vi "Puff_release2_chs.vi"() -> (5 "Plug in titles":string[](array[string]), 7 "Plug in values":string[](array[string]))   [LabVIEW 2010]
uses:
  Controls/Post_Process.ctl
  Globals/Plug_in_data_global.vi
  Globals/Meas_global.vi
  Globals/Constants_global.vi
  Globals/Dynamic_call_global.ph.vi
  <vilib>/Analysis/NI_AALPro.lvlib
panel:
  in  "PDF samples per block\n(after downsampling)":i32
  in  "Output Directory":path
  in  "Per Block Mode":T1(ring)
  in  "Averaging Samples":i32=1 min=1
  out "Valve trigger Index":dbl format="%.2f"
  out "delay":dbl format="%.2f"
  out "Pulse Width":dbl format="%.2f"
  out "falltime":dbl format="%.2f"
  out "top":dbl format="%.2f"
  out "risetime":dbl format="%.2f"
  in  "Save Time pdf?":bool
  out "Pdf":cluster{"Axis":dbl[], dbl[]}(graph)
  in  "PDF start time (s)":dbl format="%.2f"
  out "Current Block No":i32
  in  "Save averaged traces?":bool
  in  "Pause Mode":T2(ring)
  in  "OK":bool
  out "No of Valid Blocks":dbl
  out "Valve Trace":dbl[](graph)
  out "FFID Trace":cluster{dbl, dbl, dbl[]}(graph)
  out "Valve On":i32
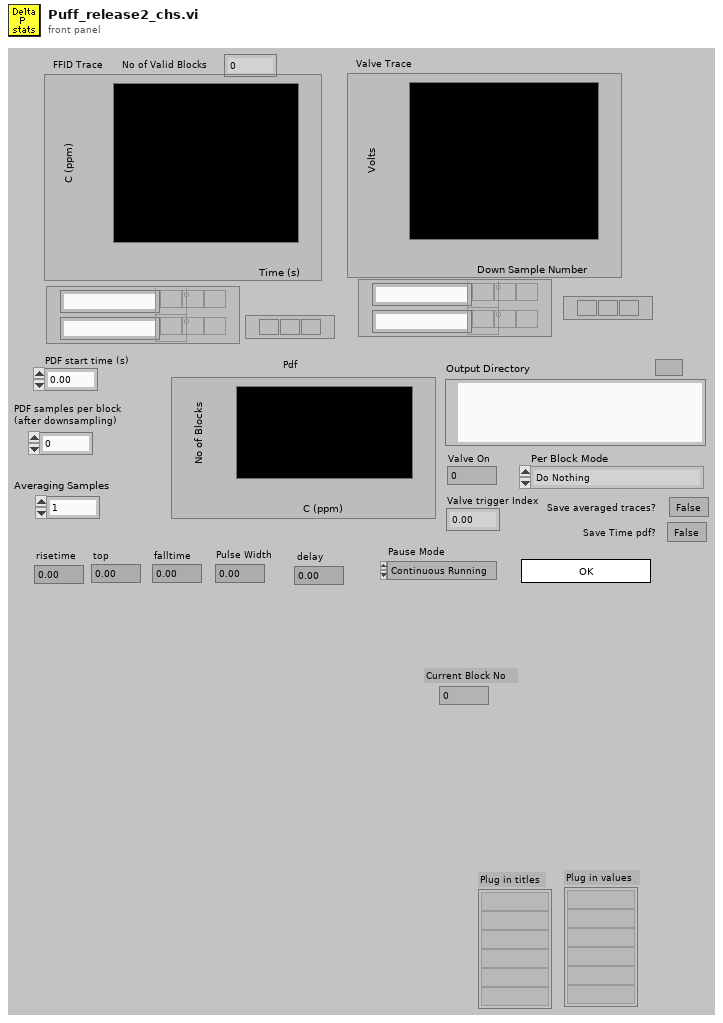
[diagram p1: front panel]
types:
  T1 = enum16{"Do Nothing", "Save Block Time Traces", "Save Jpeg plots"}
  T2 = enum16{"Continuous Running", "After Each  Block"}
  T3 = typedef "Post_Process.ctl" = enum16{"Take New Data", "Post Process Raw Data File"}
  T4 = enum32{"existing file", "new file", "new or existing file", "existing dir", "new dir", "new or existing dir", "existing file (use LLBs)", "new file (use LLBs)", "new or existing file (use LLBs)", "new or existing file or directory (use LLBs)"}
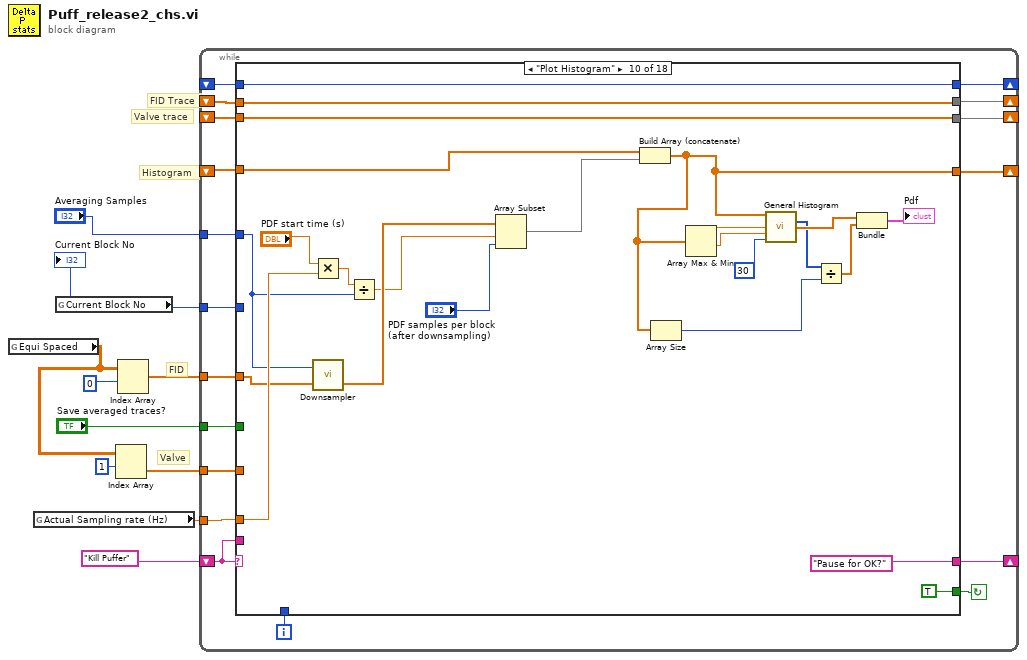
[diagram p0: block diagram]
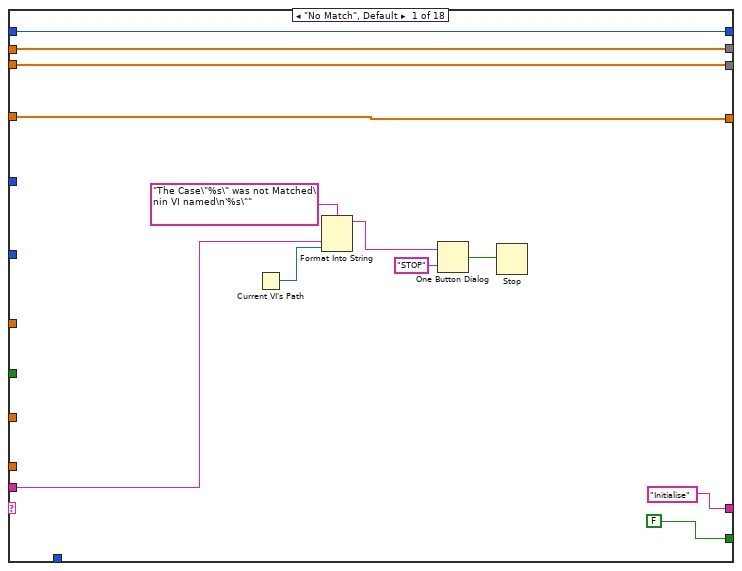
[diagram p2: hidden frame]
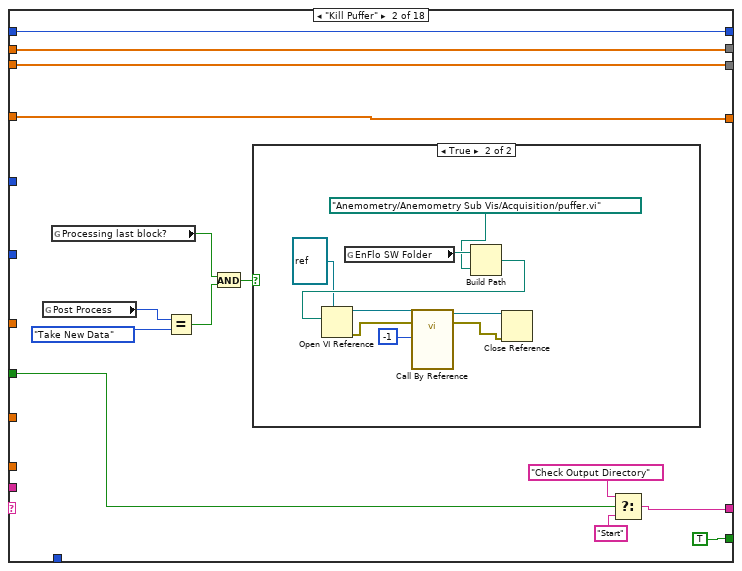
[diagram p3: hidden frame]
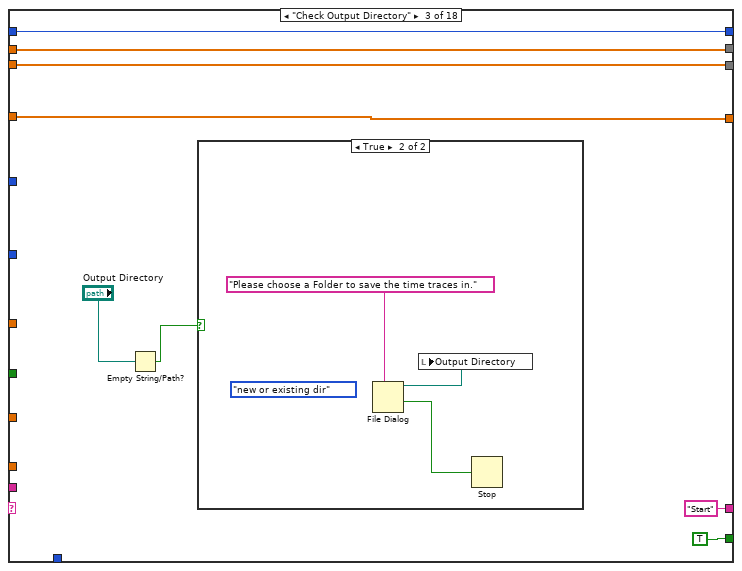
[diagram p5: hidden frame]
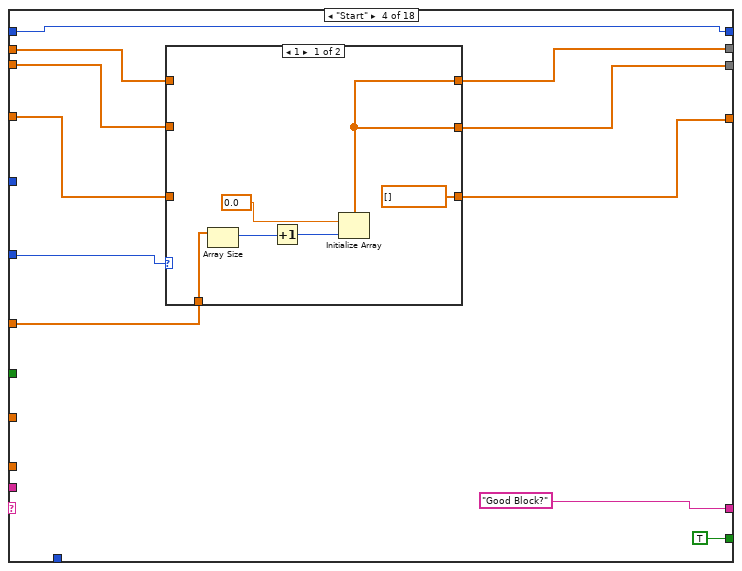
[diagram p7: hidden frame]
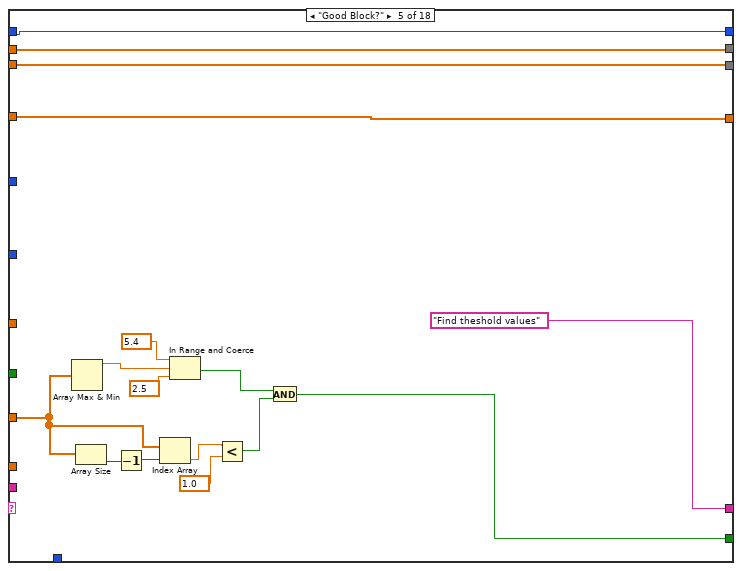
[diagram p9: hidden frame]
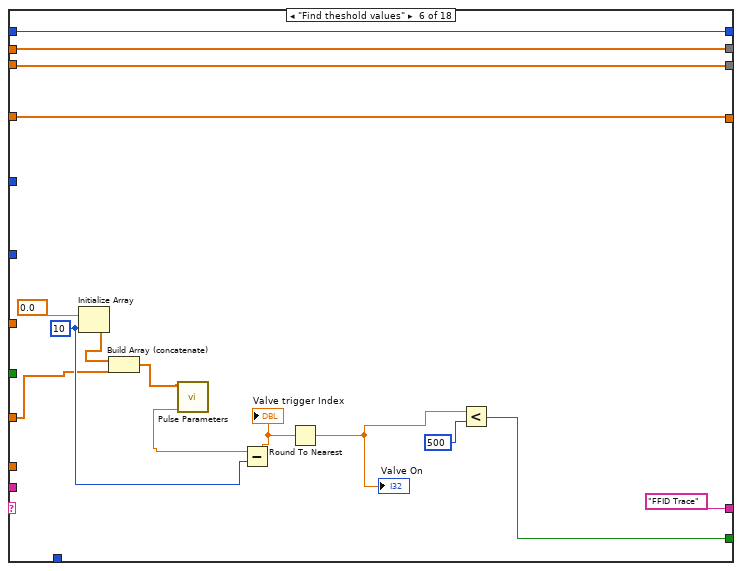
[diagram p10: hidden frame]
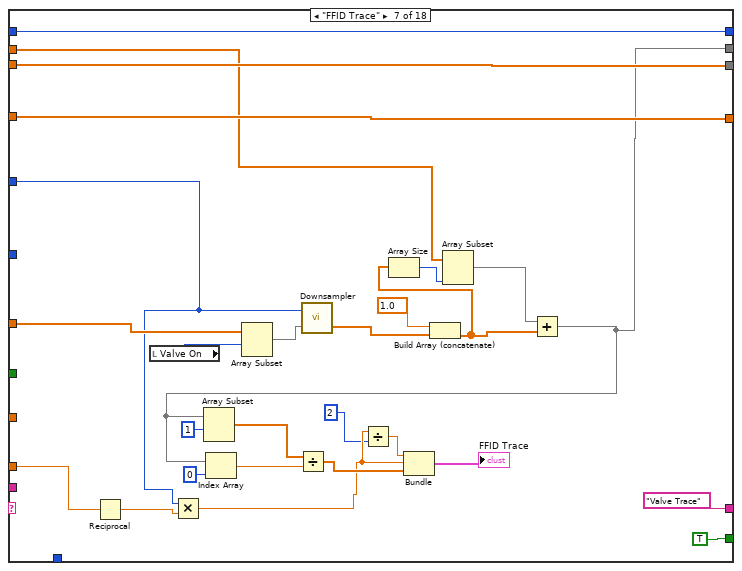
[diagram p11: hidden frame]
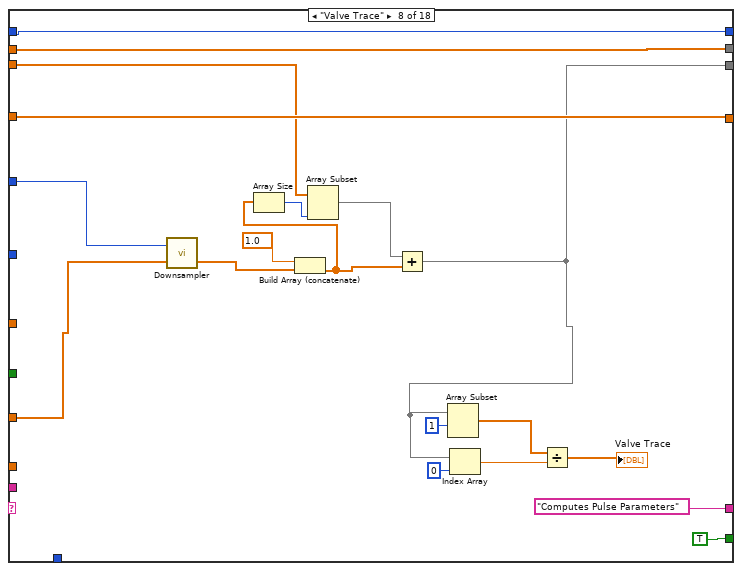
[diagram p12: hidden frame]
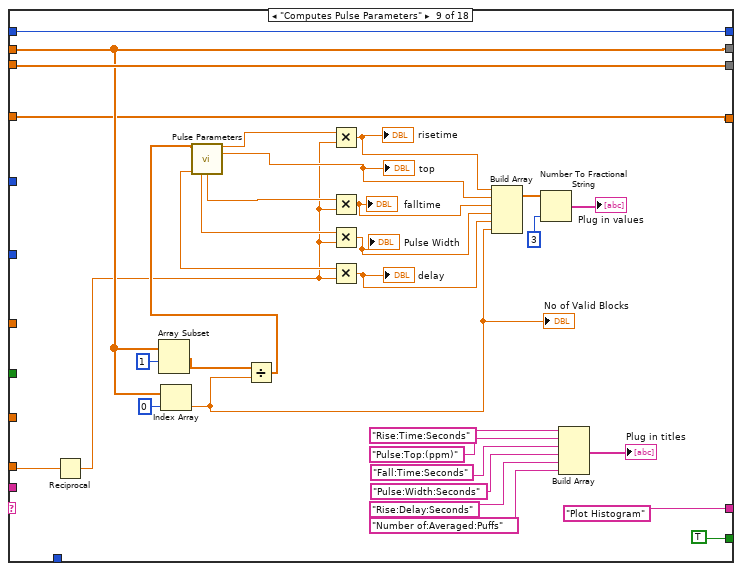
[diagram p13: hidden frame]
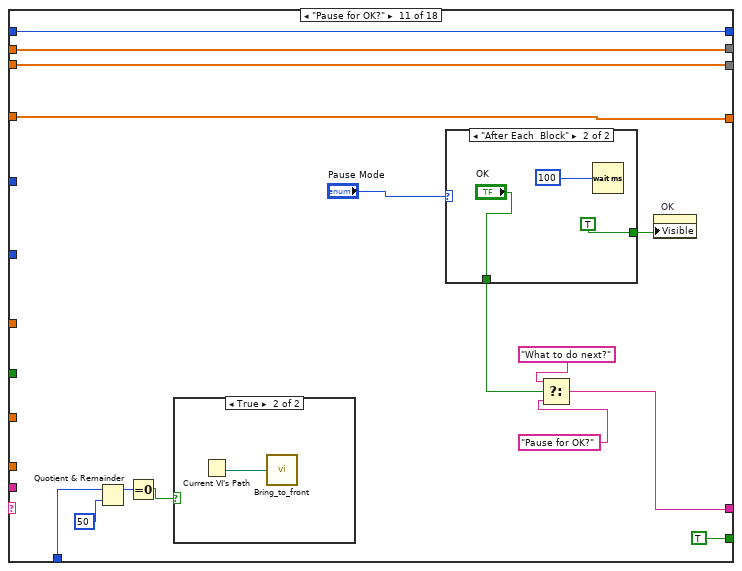
[diagram p14: hidden frame]
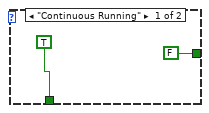
[diagram p16: hidden frame]
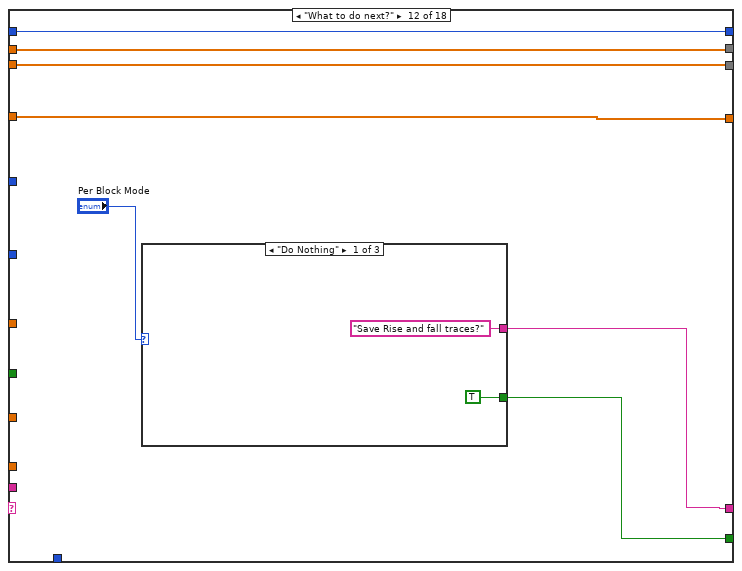
[diagram p17: hidden frame]
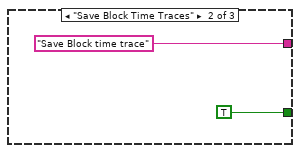
[diagram p18: hidden frame]
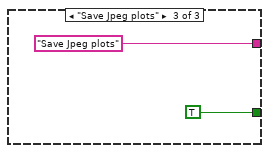
[diagram p19: hidden frame]
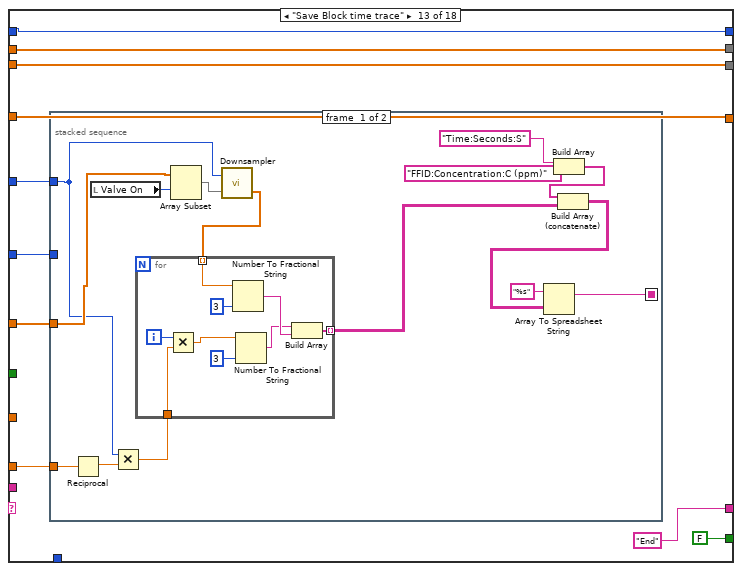
[diagram p20: hidden frame]
diagram:
  # "Valve"
  # "FID"
  # "Histogram"
  # "Valve trace"
  # "FID Trace"
  n1 = global read "Plug_in_data_global.vi" "Equi Spaced"() -> (w5:dbl[][])
  n2 = global read "Meas_global.vi" "Actual Sampling rate (Hz)"() -> (w8:dbl)
  n3 = global read "Meas_global.vi" "Current Block No"() -> (w7:i32)
  "Current Block No" <- w7
  n4 = Index Array(array=w5, index (row)=1) -> (element=w4:dbl[])  [unwired: 1 in]
  n5 = Index Array(array=w5, index (row)=0) -> (element=w9:dbl[])  [unwired: 1 in]
  n6 = while {
    shift-left: "Kill Puffer" -> [w26]
    shift-right: [w27] -> _
    shift-right: [w25] -> _
    shift-left: _ -> [w22]
    shift-right: [w24] -> _
    shift-left: _ -> [w23]
    tunnel: w9 -> [w21]
    tunnel: w8 -> [w20]
    tunnel: w7 -> [w19]
    shift-right: [w16] -> _
    shift-left: _ -> [w17]
    shift-right: [w14] -> _
    shift-left: _ -> [w15]
    tunnel: w4 -> [w13]
    tunnel: "Averaging Samples" -> [w12]
    tunnel: "Save averaged traces?" -> [w11]
    i -> [w18]
    stop <- w28 continue-if-true
    n7 = case shown="\"Plot Histogram\"" w26 {
      tunnel: [FALSE TRUE ("Processing last block?") TRUE ("Processing last block?") TRUE ("Processing last block?") w99 w121 TRUE ("Processing last block?") TRUE ("Processing last block?") TRUE ("Processing last block?") TRUE ("Processing last block?") TRUE ("Processing last block?") w249 FALSE ("Processing last block?") FALSE ("Processing last block?") w318 TRUE ("Processing last block?") "Save Time pdf?" FALSE ("Processing last block?")] -> w28
      tunnel: ["Initialise" w41 "Start" "Good Block?" "Find theshold values" "FFID Trace" "Valve Trace" "Computes Pulse Parameters" "Plot Histogram" ("f") "Pause for OK?" ("f") w230 w250 "End" "End" w320 "Save Time pdf?" "Save Time pdf" "End"] -> w27
      tunnel: w26 -> [w35 _ _ _ _ _ _ _ _ _ _ _ _ _ _ _ _ _]
      tunnel: [w32 w54 w71 w84 w110 w124 w141 w169 w174 w227 w242 w255 w271 w316 w325 w332 w407 w415] -> w25
      tunnel: [w31 w53 w70 w82 w109 w123 w150 w153 w201 w226 w241 w254 w270 w315 w324 w331 w406 w414] -> w24
      tunnel: w23 -> [w31 w53 w70 w81 w109 w123 w150 w154 w201 w226 w241 w254 w270 w315 w324 w331 w406 w414]
      tunnel: w22 -> [w32 w54 w71 w83 w110 w124 w130 w169 w174 w227 w242 w255 w271 w316 w325 w332 w407 w415]
      tunnel: w21 -> [_ _ _ w80 _ _ w149 _ _ w208 _ _ w267 w310 _ _ _ w411]
      tunnel: w20 -> [_ _ _ _ _ _ w138 _ w199 w223 _ _ w262 w307 _ _ _ _]
      tunnel: w19 -> [_ _ _ w79 _ _ _ _ _ _ _ _ w266 _ _ _ _ w410]
      tunnel: w18 -> [_ _ _ _ _ _ _ _ _ _ w239 _ _ _ _ _ _ _]
      tunnel: w17 -> [w30 w51 w67 w76 w100 w120 w146 w168 w197 w225 w235 w253 w265 w312 _ w328 _ w409]
      tunnel: [w30 w51 w67 w76 w100 w120 w146 w168 w197 w225 w235 w253 w265 w312 0 w328 0 w409] -> w16
      tunnel: w15 -> [w29 w48 w66 w77 w98 w115 w145 w163 w173 w221 w234 w252 w264 w311 w319 w327 w402 w408]
      tunnel: [w29 w48 w66 w78 w98 w115 w145 w163 w173 w213 w234 w252 w264 w311 w319 w327 w402 w408] -> w14
      tunnel: w13 -> [_ _ _ _ w95 w112 _ w156 _ _ _ _ _ _ _ _ _ _]
      tunnel: w12 -> [_ _ _ _ _ _ w135 w155 _ w205 _ _ w263 _ _ w326 _ _]
      tunnel: w11 -> [_ w44 _ _ _ _ _ _ _ _ _ _ _ _ w317 _ _ _]
      frame "No Match", Default {
        n8 = Current VI's Path() -> (path=w34:path)
        n9 = Format Into String(format string="The Case\"%s\" was not Matched\nin VI named\n'%s\"" ("Format String"), w35, w34) -> (resulting string=w38:string)  [unwired: 2 in, 1 out]
        n10 = One Button Dialog(message=w38, button name ("OK")="STOP") -> (true=w36:bool)
        n11 = Stop(stop? (T)=w36) -> ()
      }
      frame "Kill Puffer" {
        n12 = global read "Meas_global.vi" "Post Process"() -> (w50:T3)
        n13 = global read "Meas_global.vi" "Processing last block?"() -> (w46:bool)
        n14 = Equal?(x=w50, y=Post_Process."Take New Data" ("Post Process")) -> (x = y?=w47:bool)
        n15 = And(x=w46, y=w47) -> (x .and. y?=w45:bool)
        n16 = case shown="True" w45 {
          frame False {
          }
          frame True {
            n17 = global read "Constants_global.vi" "EnFlo SW Folder"() -> (w63:path)
            n18 = Build Path(base path=w63, name or relative path=path "Anemometry/Anemometry Sub Vis/Acquisition/puffer.vi") -> (appended path=w61:path)
            n19 = Open VI Reference(type specifier VI Refnum (for type only)=refnum<vi> refnum, vi path=w61) -> (vi reference=w60:refnum<vi>, error out=w56:errorcluster)  [unwired: 1 in, 3 out]
            n20 = call-by-ref "?"(reference=w60, error in=w56, "number of puffs (cont:0, stop:-1)"=-1) -> (reference out=w57:refnum<vi>, error out=w55:errorcluster)  [unwired: 2 in, 2 out]
            n21 = Close Reference(reference=w57, error in (no error)=w55) -> ()  [unwired: 1 out]
          }
        }
        n22 = Select(t="Check Output Directory", s=w44, f="Start") -> (s? t:f=w41:string)
      }
      frame "Check Output Directory" {
        n23 = Empty String/Path?(string/path="Output Directory") -> (empty?=w65:bool)
        n24 = case shown="True" w65 {
          frame False {
          }
          frame True {
            (unwired) T4."new or existing dir" ("select mode (2)")
            n25 = File Dialog(7:"Please choose a Folder to save the time traces in." ("prompt")) -> (1:w73:bool, 3:w74:path)  [unwired: 1 in, 7 out]
            n26 = local write "Output Directory"(w74) -> ()
            n27 = Stop(stop? (T)=w73) -> ()
          }
        }
      }
      frame "Start" {
        n28 = case shown="1" w79 {
          tunnel: [w87 w94] -> w84
          tunnel: w83 -> [_ w94]
          tunnel: [w87 w93] -> w82
          tunnel: w81 -> [_ w93]
          tunnel: w80 -> [w91 _]
          tunnel: [dbl[] [] w92] -> w78
          tunnel: w77 -> [_ w92]
          frame 1 {
            n29 = Array Size(array=w91) -> (size(s)=w90:i32)
            n30 = Increment(x=w90) -> (x+1=w86:i32)
            n31 = Initialize Array(0.0 ("element"), w86) -> (w87:dbl[])
          }
          frame 2, Default {
          }
        }
      }
      frame "Good Block?" {
        n32 = Array Max & Min(array=w95) -> (max value=w97:dbl)  [unwired: 3 out]
        n33 = Array Size(array=w95) -> (size(s)=w106:i32)
        n34 = Decrement(x=w106) -> (x-1=w105:i32)
        n35 = Index Array(array=w95, index=w105) -> (element=w104:dbl)
        n36 = In Range and Coerce(upper limit=5.4, x=w97, lower limit=2.5 ("y")) -> (In Range?=w101:bool)  [unwired: 1 out]
        n37 = Less?(x=w104, y=1.0) -> (x < y?=w102:bool)
        n38 = And(x=w101, y=w102) -> (x .and. y?=w99:bool)
      }
      frame "Find theshold values" {
        w116 = 10 ("dimension size")
        n39 = Initialize Array(0.0, w116) -> (w117:dbl[])
        n40 = Build Array (concatenate)(w117, w112) -> (w118:dbl[])
        n41 = call <vilib>:"Pulse Parameters.vi"("X"=w118) -> ("delay"=w114:dbl)  [unwired: 14 out]
        n42 = Subtract(x=w114, y=w116) -> (x-y=w113:dbl)
        "Valve trigger Index" <- w113
        n43 = Round To Nearest(number=w113) -> (nearest integer value=w111:dbl)
        "Valve On" <- w111
        n44 = Less?(x=w111, y=500) -> (x < y?=w121:bool)
      }
      frame "FFID Trace" {
        n45 = Reciprocal(x=w138) -> (1/x=w134:dbl)
        n46 = local read "Valve On"() -> (w147:i32)
        n47 = Multiply(x=w135, y=w134) -> (x*y=w128:dbl)
        n48 = Array Subset(array=w149, index=w147) -> (w136:dbl[])  [unwired: 1 in]
        n49 = call "Downsampler.vi"("Input Array"=w136, "Averaging samples"=w135) -> ("Downsampled Array"=w133:dbl[])  [unwired: 1 out]
        n50 = Divide(x=w128, y=2) -> (x/y=w126:dbl)
        n51 = Build Array (concatenate)(1.0, w133) -> (w131:dbl[])
        n52 = Array Size(array=w131) -> (size(s)=w132:i32)
        n53 = Array Subset(array=w130, length=w132) -> (w129:dbl[])  [unwired: 1 in]
        n54 = Add(x=w129, y=w131) -> (x+y=w141:dbl[])
        n55 = Array Subset(array=w141, index=1) -> (w140:dbl[])  [unwired: 1 in]
        n56 = Index Array(array=w141, index=0) -> (element=w139:dbl)
        n57 = Divide(x=w140, y=w139) -> (x/y=w144:dbl[])
        n58 = Bundle(w126, w128, w144) -> (→"FFID Trace":cluster{dbl, dbl, dbl[]})  [unwired: 1 out]
      }
      frame "Valve Trace" {
        n59 = call "Downsampler.vi"("Input Array"=w156, "Averaging samples"=w155) -> ("Downsampled Array"=w160:dbl[])  [unwired: 1 out]
        n60 = Build Array (concatenate)(1.0, w160) -> (w158:dbl[])
        n61 = Array Size(array=w158) -> (size(s)=w159:i32)
        n62 = Array Subset(array=w154, length=w159) -> (w157:dbl[])  [unwired: 1 in]
        n63 = Add(x=w157, y=w158) -> (x+y=w153:dbl[])
        n64 = Array Subset(array=w153, index=1) -> (w165:dbl[])  [unwired: 1 in]
        n65 = Index Array(array=w153, index=0) -> (element=w164:dbl)
        n66 = Divide(x=w165, y=w164) -> (x/y=→"Valve Trace":dbl[])
      }
      frame "Computes Pulse Parameters" {
        n67 = Reciprocal(x=w199) -> (1/x=w172:dbl)
        n68 = Array Subset(array=w174, index=1) -> (w177:dbl[])  [unwired: 1 in]
        n69 = Index Array(array=w174, index=0) -> (element=w176:dbl)
        "No of Valid Blocks" <- w176
        n70 = Divide(x=w177, y=w176) -> (x/y=w175:dbl[])
        n71 = call <vilib>:"Pulse Parameters.vi"("X"=w175) -> ("risetime"=w196:dbl, "top"=w182:dbl, "delay"=w193:dbl, "duration"=w194:dbl, "falltime"=w195:dbl)  [unwired: 10 out]
        "top" <- w182
        n72 = Multiply(x=w196, y=w172) -> (x*y=w181:dbl)
        "risetime" <- w181
        n73 = Multiply(x=w195, y=w172) -> (x*y=w180:dbl)
        "falltime" <- w180
        n74 = Multiply(x=w194, y=w172) -> (x*y=w179:dbl)
        "Pulse Width" <- w179
        n75 = Multiply(x=w193, y=w172) -> (x*y=w178:dbl)
        "delay" <- w178
        n76 = Build Array(w181, w182, w180, w179, w178, w176) -> (w192:dbl[])
        n77 = Number To Fractional String(number=w192, precision (6)=i16 3) -> (F-format string=→"Plug in values":string[])  [unwired: 2 out]
        n78 = Build Array("Rise:Time:Seconds", "Pulse:Top:(ppm)", "Fall:Time:Seconds", "Pulse:Width:Seconds", "Rise:Delay:Seconds", "Number of:Averaged:Puffs") -> (→"Plug in titles":string[])
      }
      frame "Plot Histogram" {
        n79 = Multiply(x="PDF start time (s)", y=w223) -> (x*y=w206:dbl)
        n80 = call "Downsampler.vi"("Input Array"=w208, "Averaging samples"=w205) -> ("Downsampled Array"=w207:dbl[])  [unwired: 1 out]
        n81 = Divide(x=w206, y=w205) -> (x/y=w204:dbl)
        n82 = Array Subset(array=w207, index=w204, length="PDF samples per block\n(after downsampling)") -> (w222:dbl[])
        n83 = Build Array (concatenate)(w221, w222) -> (w213:dbl[])
        n84 = Array Size(array=w213) -> (size(s)=w211:i32)
        n85 = Array Max & Min(array=w213) -> (max value=w220:dbl, min value=w219:dbl)  [unwired: 2 out]
        n86 = call <vilib>:"General Histogram.vi"("X"=w213, "max"=w220, "min"=w219, "# bins"=30) -> ("Histogram"=w212:i32[], "Axis"=w217:dbl[])  [unwired: 2 in, 8 out]
        n87 = Divide(x=w212, y=w211) -> (x/y=w209:dbl[])
        n88 = Bundle("Axis"=w217, w209) -> (→"Pdf":cluster{"Axis":dbl[], dbl[]})  [unwired: 1 out]
      }
      frame "Pause for OK?" {
        n89 = Quotient & Remainder(x=w239, y=50) -> (x-y*floor(x/y)=w237:i32)  [unwired: 1 out]
        n90 = Equal To 0?(x=w237) -> (x = 0?=w236:bool)
        n91 = case shown="True" w236 {
          frame False {
          }
          frame True {
            n92 = Current VI's Path() -> (path=w243:path)
            n93 = call "Bring_to_front.vi"("path"=w243) -> ()
          }
        }
        n94 = case shown="\"After Each  Block\"" "Pause Mode" {
          tunnel: [TRUE "OK"] -> w231
          tunnel: [FALSE TRUE] -> w240
          frame "Continuous Running" {
          }
          frame "After Each  Block" {
            n95 = Wait (ms)(milliseconds to wait=u32 100 ("f")) -> ()  [unwired: 1 out]
          }
        }
        n96 = Select(t="What to do next?" ("f"), s=w231, f="Pause for OK?") -> (s? t:f=w230:string)
        n97 = property on="OK" class="Bool"("Visible"=w240) -> ()  [unwired: 2 in, 2 out]
      }
      frame "What to do next?" {
        n98 = case shown="\"Do Nothing\"" "Per Block Mode" {
          tunnel: ["Save Rise and fall traces?" ("t") "Save Block time trace" ("t") "Save Jpeg plots" ("t")] -> w250
          tunnel: [TRUE TRUE TRUE] -> w249
          frame "Do Nothing" {
          }
          frame "Save Block Time Traces" {
          }
          frame "Save Jpeg plots" {
          }
        }
      }
      frame "Save Block time trace" {
        n99 = stacked-sequence {
          seq-local: [w281 _] -> [_ w301]
          tunnel: w267 -> [w278 _]
          tunnel: w266 -> [_ w299]
          tunnel: w263 -> [w273 _]
          tunnel: w262 -> [w275 _]
          frame #0 {
            n100 = Reciprocal(x=w275) -> (1/x=w274:dbl)
            n101 = local read "Valve On"() -> (w279:i32)
            n102 = Multiply(x=w273, y=w274) -> (x*y=w272:dbl)
            n103 = Array Subset(array=w278, index=w279) -> (w277:dbl[])  [unwired: 1 in]
            n104 = call "Downsampler.vi"("Input Array"=w277, "Averaging samples"=w273) -> ("Downsampled Array"=w276:dbl[])  [unwired: 1 out]
            n105 = for {
              tunnel: [w293] -> w280 mode=indexing
              tunnel: w276 -> [w290] mode=indexing
              tunnel: w272 -> [w289]
              i -> [w288]
              n106 = Multiply(x=w288, y=w289) -> (x*y=w287:dbl)
              n107 = Number To Fractional String(number=w290, precision (6)=i16 3) -> (F-format string=w292:string)  [unwired: 2 out]
              n108 = Number To Fractional String(number=w287, precision (6)=i16 3) -> (F-format string=w291:string)  [unwired: 2 out]
              n109 = Build Array(w291, w292) -> (w293:string[])
            }
            n110 = Build Array("Time:Seconds:S", "FFID:Concentration:C (ppm)") -> (w284:string[])
            n111 = Build Array (concatenate)(w284, w280) -> (w283:string[][])
            n112 = Array To Spreadsheet String(array=w283, 3:"%s" ("format string")) -> (spreadsheet string=w281:string)  [unwired: 1 out]
          }
          frame #1 {
            w303 = TRUE  # advisory dialog? (display:T)
            n113 = global read "Meas_global.vi" "Raw data file"() -> (w306:path)
            n114 = Strip Path(path=w306) -> (name=w300:string)  [unwired: 1 out]
            n115 = local read "Output Directory"() -> (w296:path)
            n116 = Format Into String(format string="_B%d", initial string=w300, w299) -> (resulting string=w297:string)  [unwired: 1 in, 1 out]
            n117 = Build Path(base path=w296, name or relative path=w297) -> (appended path=w305:path)
            n118 = call "Find_Unique_Filename.vi"("Path In"=w305) -> ("Unique Path Out"=w304:path)  [unwired: 1 in, 1 out]
            n119 = call "Write_Characters_To_File.vi"("file path (dialog if empty)"=w304, "advisory dialog? (display:T)"=w303, "character string"=w301, "append to file? (new file:F)"=FALSE) -> ()  [unwired: 1 in, 4 out]
          }
        }
      }
      frame "Save Jpeg plots" {
        n120 = local read "Valve On"() -> (w309:i32)
        n121 = Array Subset(array=w310, index=w309) -> (w308:dbl[])  [unwired: 1 in]
        n122 = call "Puff_realisation_display.vi"("Actual Sampling rate (Hz)"=w307, "Input Array"=w308) -> ()  [unwired: 2 out]
      }
      frame "Save Rise and fall traces?" {
        n123 = Select(t="Save averaged time trace", s=w317, f="Save Time PDF?") -> (s? t:f=w320:string)
        n124 = global read "Meas_global.vi" "Processing last block?"() -> (w318:bool)
      }
      frame "Save averaged time trace" {
        n125 = stacked-sequence {
          seq-local: [w345 _] -> [_ w380]
          tunnel: w326 -> [w335 _]
          frame #0 {
            n126 = local read "FFID Trace"() -> (w354:cluster{dbl, dbl, dbl[]})
            n127 = local read "Valve On"() -> (w334:i32)
            n128 = local read "Valve Trace"() -> (w338:dbl[])
            n129 = Unbundle(w354) -> (w352:dbl, w353:dbl, w336:dbl[])
            n130 = Divide(x=w334, y=w335) -> (x/y=w333:dbl)
            n131 = Array Subset(array=w338, index=w333) -> (w337:dbl[])  [unwired: 1 in]
            n132 = for {
              tunnel: w353 -> [w365]
              tunnel: w352 -> [w364]
              tunnel: w336 -> [w359] mode=indexing
              tunnel: [w362] -> w350 mode=indexing
              tunnel: w337 -> [w360] mode=indexing
              i -> [w366]
              n133 = Multiply(x=w365, y=w366) -> (x*y=w363:dbl)
              n134 = Add(x=w364, y=w363) -> (x+y=w361:dbl)
              n135 = Build Array(w361, w360, w359) -> (w362:dbl[])
            }
            n136 = Build Array("Time:(s):T=0 when valve opened", "Source:Valve:Voltage", "FFID:Concentration:C") -> (w342:string[])
            n137 = for {
              tunnel: w342 -> [w358] mode=indexing
              tunnel: [w357] -> w341 mode=indexing
              tunnel: [w356] -> w340 mode=indexing
              tunnel: [w355] -> w339 mode=indexing
              n138 = call "Split_Ch_name.vi"("Ch name"=w358) -> ("Top level"=w357:string, "Middle"=w356:string, "Low level"=w355:string)
            }
            n139 = Number To Fractional String(number=w350, precision (6)=i16 3) -> (F-format string=w349:string[][])  [unwired: 2 out]
            n140 = Build Array (concatenate)(w341, w340, w339, w349) -> (w347:string[][])
            n141 = Array To Spreadsheet String(array=w347, 3:"%s" ("format string")) -> (spreadsheet string=w345:string)  [unwired: 1 out]
          }
          frame #1 {
            w392 = TRUE  # advisory dialog? (display:T)
            n142 = local read "No of Valid Blocks"() -> (w368:dbl)
            n143 = global read "Meas_global.vi" "Raw data file"() -> (w397:path)
            n144 = global read "Dynamic_call_global.ph.vi" "Plug in titles"() -> (w373:string[])
            n145 = global read "Dynamic_call_global.ph.vi" "Plug in values"() -> (w370:string[])
            n146 = Strip Path(path=w397) -> (name=w378:string)  [unwired: 1 out]
            n147 = String Subset(string=w378, offset (0)=0, length (rest)=28 ("length (rest)")) -> (substring=w375:string)
            n148 = Number To Decimal String(number=w368) -> (decimal integer string=w367:string)  [unwired: 1 out]
            n149 = Build Array (concatenate)("No of:Blocks:Processed", w373) -> (w371:string[])
            n150 = Build Array (concatenate)(w367, w370) -> (w369:string[])
            n151 = local read "Output Directory"() -> (w374:path)
            n152 = for {
              tunnel: w371 -> [w401] mode=indexing
              tunnel: [w400] -> w390 mode=indexing
              tunnel: [w399] -> w389 mode=indexing
              tunnel: [w398] -> w388 mode=indexing
              n153 = call "Split_Ch_name.vi"("Ch name"=w401) -> ("Top level"=w400:string, "Middle"=w399:string, "Low level"=w398:string)
            }
            n154 = Concatenate Strings(w375, "_P" ("string")) -> (w396:string)
            n155 = Initialize Array("", 15) -> (w385:string[])
            n156 = Build Path(base path=w374, name or relative path=w396) -> (appended path=w394:path)
            n157 = call "Asterisk_header.vi"("Channel names"=w385) -> ("Header string"=w381:string)
            n158 = call "Find_Unique_Filename.vi"("Path In"=w394) -> ("Unique Path Out"=w393:path)  [unwired: 1 in, 1 out]
            n159 = Build Array(w390, w389, w388, w369) -> (w386:string[][])
            n160 = Array To Spreadsheet String(array=w386, 3:"%s" ("format string")) -> (spreadsheet string=w382:string)  [unwired: 1 out]
            n161 = Concatenate Strings(w382, w381, w380) -> (w379:string)
            n162 = call "Write_Characters_To_File.vi"("file path (dialog if empty)"=w393, "advisory dialog? (display:T)"=w392, "character string"=w379, "append to file? (new file:F)"=FALSE) -> ()  [unwired: 1 in, 4 out]
          }
        }
      }
      frame "Save Time pdf?" {
      }
      frame "Save Time pdf" {
        n163 = stacked-sequence {
          seq-local: [w426 _] -> [_ w459]
          tunnel: w411 -> [_ _]
          tunnel: w410 -> [_ _]
          frame #0 {
            n164 = local read "Pdf"() -> (w424:cluster{"Axis":dbl[], dbl[]})
            n165 = Unbundle(w424) -> ("Axis"=w423:dbl[], w422:dbl[])
            n166 = for {
              tunnel: w422 -> [w437] mode=indexing
              tunnel: w423 -> [w444] mode=indexing
              tunnel: [w443] -> w425 mode=indexing
              shift-right: [w436] -> _
              shift-left: 0.0 -> [w438]
              n167 = Add(x=w437, y=w438) -> (x+y=w436:dbl)
              n168 = Number To Fractional String(number=w437, precision (6)=i16 3) -> (F-format string=w441:string)  [unwired: 2 out]
              n169 = Number To Fractional String(number=w436, precision (6)=i16 3) -> (F-format string=w435:string)  [unwired: 2 out]
              n170 = Number To Fractional String(number=w444, precision (6)=i16 3) -> (F-format string=w442:string)  [unwired: 2 out]
              n171 = Build Array(w442, w441, w435) -> (w443:string[])
            }
            n172 = Build Array("FFID:Concentration:C (ppm)", "Pdf:Bin:Frequency", "Cumulative Pdf:Bin:Frequency") -> (w421:string[])
            n173 = for {
              tunnel: w421 -> [w434] mode=indexing
              tunnel: [w433] -> w420 mode=indexing
              tunnel: [w432] -> w419 mode=indexing
              tunnel: [w431] -> w418 mode=indexing
              n174 = call "Split_Ch_name.vi"("Ch name"=w434) -> ("Top level"=w433:string, "Middle"=w432:string, "Low level"=w431:string)
            }
            n175 = Build Array (concatenate)(w420, w419, w418, w425) -> (w428:string[][])
            n176 = Array To Spreadsheet String(array=w428, 3:"%s" ("format string")) -> (spreadsheet string=w426:string)  [unwired: 1 out]
          }
          frame #1 {
            w474 = TRUE  # advisory dialog? (display:T)
            n177 = global read "Dynamic_call_global.ph.vi" "Plug in titles"() -> (w448:string[])
            n178 = global read "Dynamic_call_global.ph.vi" "Plug in values"() -> (w450:string[])
            n179 = local read "No of Valid Blocks"() -> (w452:dbl)
            n180 = global read "Meas_global.vi" "Raw data file"() -> (w477:path)
            n181 = local read "PDF start time (s)"() -> (w470:dbl)
            n182 = Strip Path(path=w477) -> (name=w455:string)  [unwired: 1 out]
            n183 = Build Array (concatenate)("No of:Blocks:Processed", w448) -> (w447:string[])
            n184 = Number To Decimal String(number=w452) -> (decimal integer string=w451:string)  [unwired: 1 out]
            n185 = Build Array (concatenate)(w451, w450) -> (w449:string[])
            n186 = String Subset(string=w455, offset (0)=0, length (rest)=20 ("length (rest)")) -> (substring=w454:string)
            n187 = for {
              tunnel: w447 -> [w481] mode=indexing
              tunnel: [w480] -> w469 mode=indexing
              tunnel: [w479] -> w468 mode=indexing
              tunnel: [w478] -> w467 mode=indexing
              n188 = call "Split_Ch_name.vi"("Ch name"=w481) -> ("Top level"=w480:string, "Middle"=w479:string, "Low level"=w478:string)
            }
            n189 = Format Into String(format string="_T=%d", initial string=w454, w470) -> (resulting string=w471:string)  [unwired: 1 in, 1 out]
            n190 = local read "Output Directory"() -> (w453:path)
            n191 = Initialize Array("", 15) -> (w464:string[])
            n192 = Build Path(base path=w453, name or relative path=w471) -> (appended path=w476:path)
            n193 = call "Asterisk_header.vi"("Channel names"=w464) -> ("Header string"=w460:string)
            n194 = call "Find_Unique_Filename.vi"("Path In"=w476) -> ("Unique Path Out"=w475:path)  [unwired: 1 in, 1 out]
            n195 = Build Array(w469, w468, w467, w449) -> (w465:string[][])
            n196 = Array To Spreadsheet String(array=w465, 3:"%s" ("format string")) -> (spreadsheet string=w461:string)  [unwired: 1 out]
            n197 = Concatenate Strings(w461, w460, w459) -> (w458:string)
            n198 = call "Write_Characters_To_File.vi"("file path (dialog if empty)"=w475, "advisory dialog? (display:T)"=w474, "character string"=w458, "append to file? (new file:F)"=FALSE) -> ()  [unwired: 1 in, 4 out]
          }
        }
      }
    }
  }
